vi "Generate Trigger Signal.vi"(7 "Mode (T: Initiate)":bool=TRUE, 8 "Error In (no error)":errorcluster, 10 "Channel (1)":i32=1, 11 "VISA Resource Name":refnum<visa-resource-name>) -> (0 "Error Out":errorcluster, 3 "VISA Resource Name Out":refnum<visa-resource-name>)   [LabVIEW 2018, in "Agilent PNA Series.lvlib"]
doc: "This VI generates or stops trigger signal."
uses:
  Agilent PNA Series.lvlib
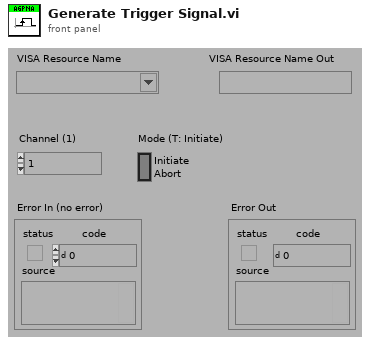
[diagram p1: front panel]
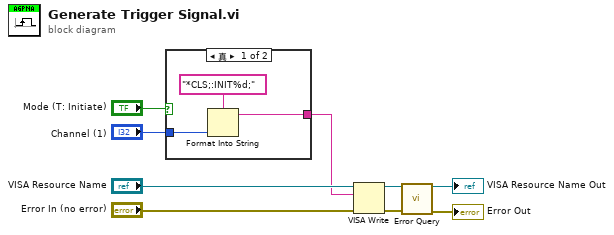
[diagram p0: block diagram]
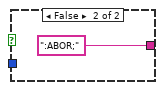
[diagram p2: hidden frame]
diagram:
  n1 = case shown="真" "Mode (T: Initiate)" {
    tunnel: "Channel (1)" -> [w10 _]
    tunnel: [w11 ":ABOR;" ("format string")] -> w5
    frame True {
      n2 = Format Into String(format string="*CLS;:INIT%d;", w10) -> (resulting string=w11:string)  [unwired: 2 in, 1 out]
    }
    frame False {
    }
  }
  n3 = VISA Write(VISA resource name="VISA Resource Name", write buffer=w5, error in (no error)="Error In (no error)") -> (VISA resource name out=w4:refnum<visa-resource-name>, error out=w3:errorcluster)  [unwired: 1 out]
  n4 = call "Error Query.vi"("VISA Resource Name"=w4, "error in (no error)"=w3) -> ("VISA Resource Name Out"=→"VISA Resource Name Out":refnum<visa-resource-name>, "error out"=→"Error Out":errorcluster)  [unwired: 10 in, 2 out]
